vi "TestData_MySQL_OP-TEST.vi"(8 "error in (no error)":errorcluster, 10 "SQL File":path, 11 "Connection In":refnum<k7>) -> (0 "error out":errorcluster, 2 "ok?":bool, 3 "ADODB._Connection Out":refnum<k7>)   [LabVIEW 2012, in "Lib_UEL.ATE.lvlib" / "Lib_TestData.lvlib"]
uses:
  Lib_TestData.lvlib
  <vilib>/Utility/file.llb/Read From Spreadsheet File (string).vi
  <vilib>/Utility/file.llb/Write To Spreadsheet File (string).vi
panel:
  out "数组":i32[](array[numeric])
  out "Data":string[][](array[string])
  in  "Output Failed Record":bool
  out "Modified?":bool
  in  "Comment Signal":string
  out "Result":T1
  in  "TXT File In":path
  in  "ConnectionString":T2={"IP"="localhost", "Port"="3306", "DataBase"="uel_te", "User"="root", "Password"="alpha130723"}
  out "结果字符串":string
  # "功能描述:\n- 批量插入文本数据记录到数据库.\n- 插入成功的记录, 记录前以';'注释\n- 插入失败的记录, 不注释\n- 已注释的记录, 不会进行插入数据的操作.\n- Output Failed Record开关: 失败的记录是否导出到一个单独的文件, 打开后, 输出到文件名: 原文件名+FailInsert+Date."
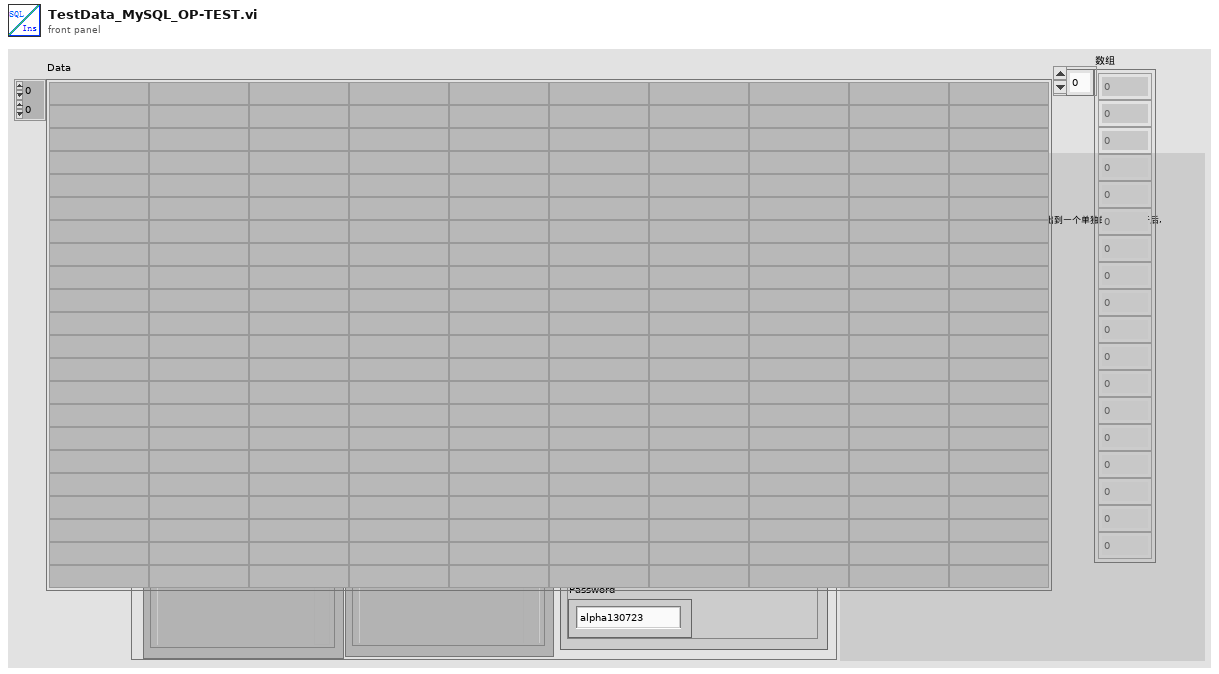
[diagram p1: front panel]
types:
  T1 = cluster{"Total":u32, "NG":u32, "OK":u32, "Ignore":u32}
  T2 = cluster{"IP":string, "Port":string, "DataBase":string, "User":string, "Password":string}
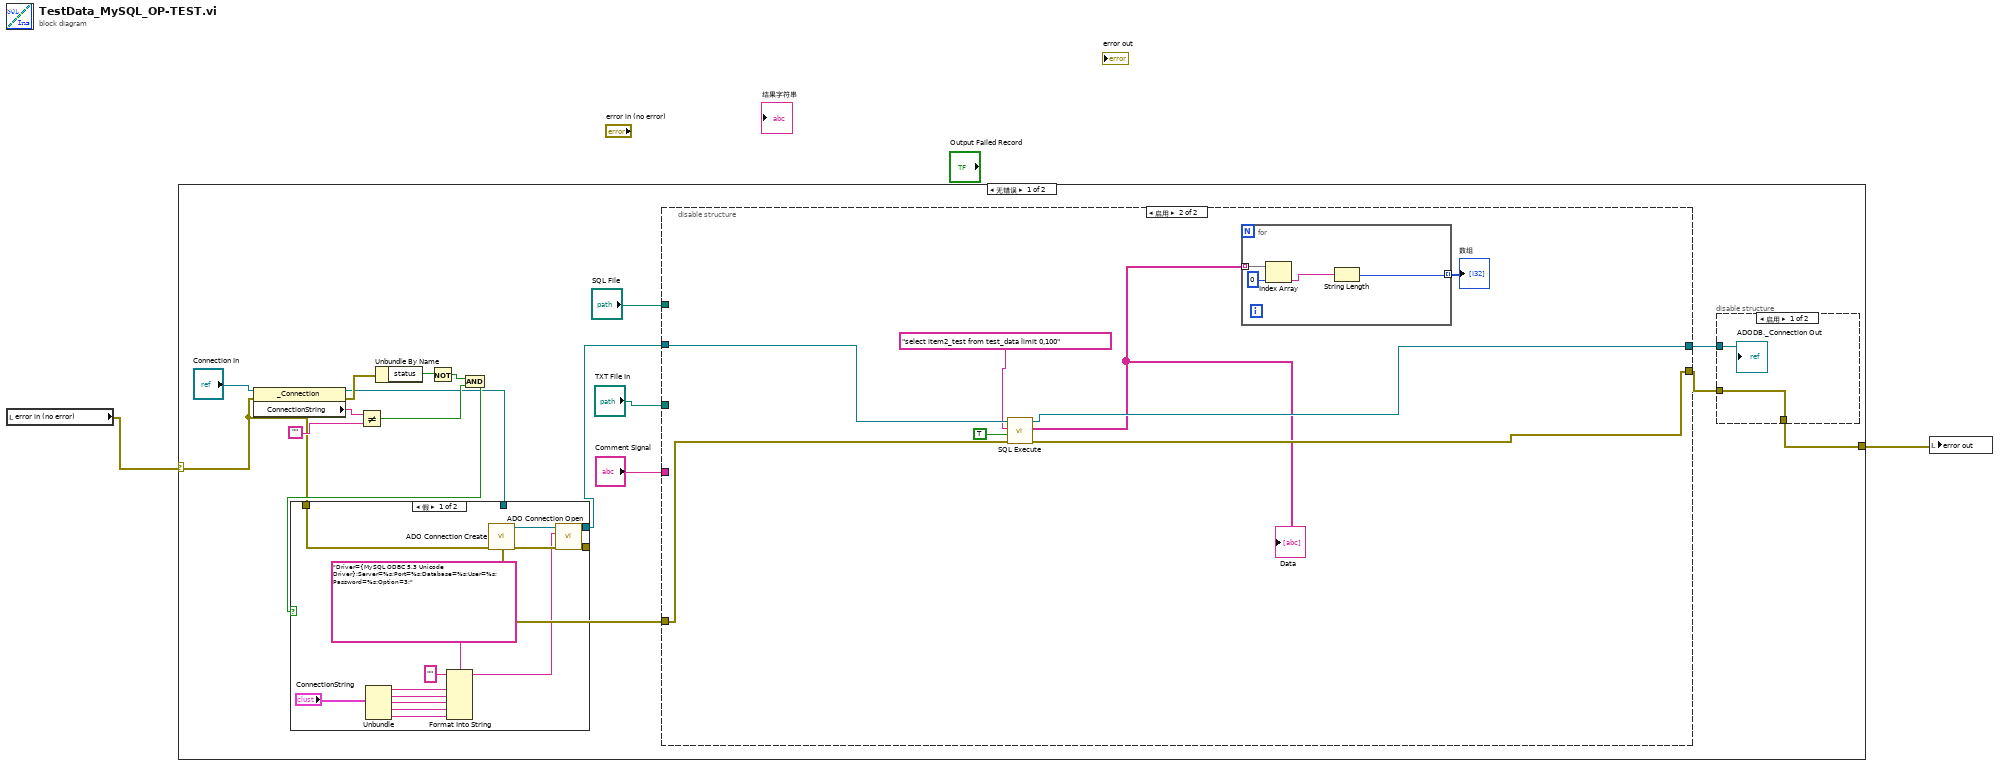
[diagram p0: block diagram]
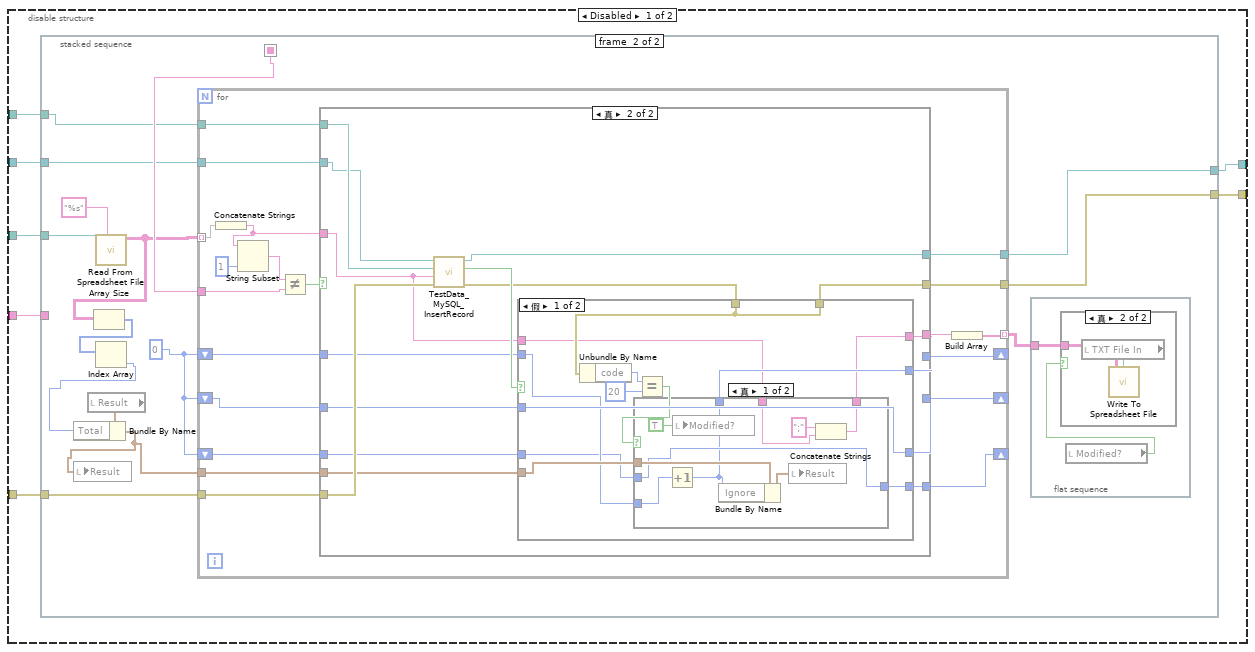
[diagram p2: hidden frame]
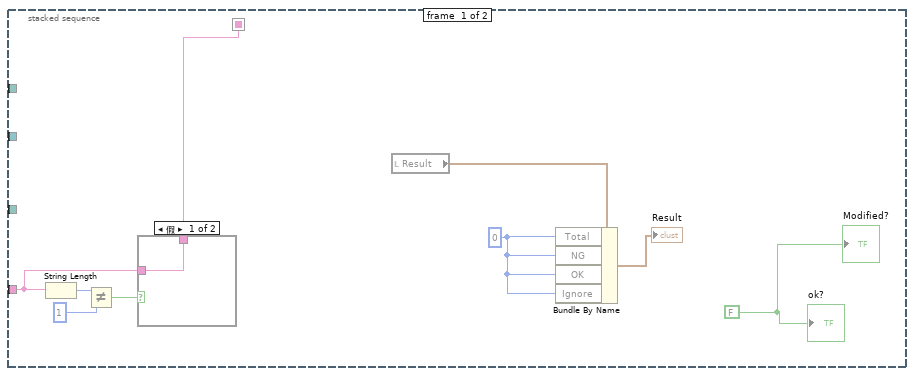
[diagram p3: hidden frame]
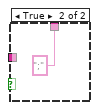
[diagram p4: hidden frame]
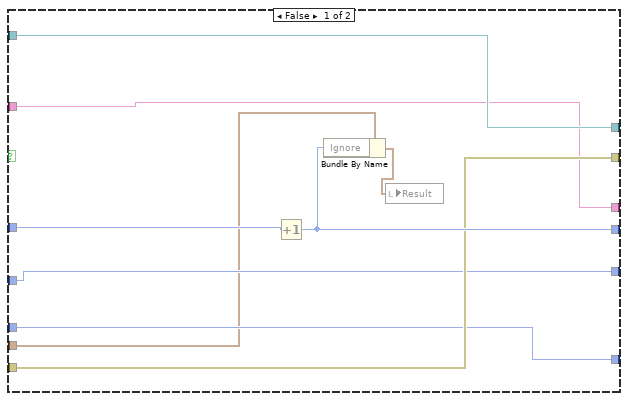
[diagram p6: hidden frame]
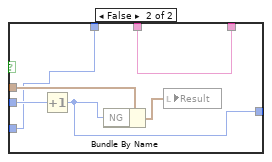
[diagram p7: hidden frame]
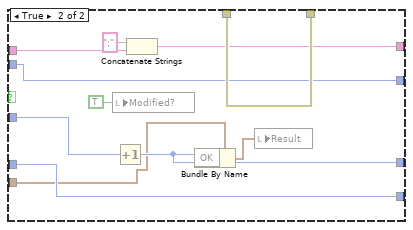
[diagram p8: hidden frame]
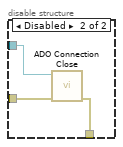
[diagram p10: hidden frame]
diagram:
  n1 = local read "error in (no error)"() -> (w1:errorcluster)
  n2 = case shown="无错误" w1 {
    selector: w1 -> [w3 w174]
    tunnel: [w4 w174] -> w2
    frame No Error {
      n3 = property class="_Connection"(reference="Connection In", error in=w3) -> (reference out=w6:refnum<k7>, error out=w11:errorcluster, "ConnectionString"=w13:string)
      n4 = Not Equal?(x=w13, y="") -> (x != y?=w8:bool)
      n5 = Unbundle By Name(w11) -> ("status"=w10:bool)
      n6 = Not(x=w10) -> (.not. x?=w9:bool)
      n7 = And(x=w9, y=w8) -> (x .and. y?=w7:bool)
      n8 = case shown="假" w7 {
        tunnel: [w166 w168] -> w15
        tunnel: w6 -> [_ w168]
        tunnel: w3 -> [w154 w167]
        tunnel: [w153 w167] -> w5
        frame False {
          n9 = Unbundle("ConnectionString") -> ("IP"=w158:string, "Port"=w159:string, "DataBase"=w160:string, "User"=w161:string, "Password"=w162:string)
          n10 = Format Into String(format string="Driver={MySQL ODBC 5.3 Unicode Driver};Server=%s;Port=%s;Database=%s;User=%s; Password=%s;Option=3;" ("格式字符串"), initial string="" ("初始字符串"), w158, w159, w160, w161, w162) -> (resulting string=w164:string)  [unwired: 1 in, 1 out]
          n11 = call <userlib>:"ADO Connection Create.vi"("error in (no error)"=w154) -> ("error out"=w163:errorcluster, "ADODB._Connection Out"=w165:refnum<k7>)  [unwired: 9 in]
          n12 = call <userlib>:"ADO Connection Open.vi"("error in (no error)"=w163, "ConnectionString"=w164, "ADODB._Connection In"=w165) -> ("error out"=w153:errorcluster, "ADODB._Connection Out"=w166:refnum<k7>)  [unwired: 7 in]
        }
        frame True {
        }
      }
      n13 = disable-structure shown="启用" {
        disable-tunnel: [w27 w145] -> w20
        disable-tunnel: "SQL File" -> [w26 _]
        disable-tunnel: "TXT File In" -> [w25 _]
        disable-tunnel: "Comment Signal" -> [w24 _]
        disable-tunnel: [w23 w144] -> w16
        disable-tunnel: w15 -> [w22 w147]
        disable-tunnel: w5 -> [w21 w146]
        frame Disabled {
          n14 = stacked-sequence {
            seq-local: [w33 _] -> [_ w51]
            tunnel: w21 -> [_ w47]
            tunnel: [_ w44] -> w27
            tunnel: [_ w45] -> w23
            tunnel: w26 -> [_ w46]
            tunnel: w25 -> [_ w53]
            tunnel: w24 -> [w32 _]
            tunnel: w22 -> [_ w43]
            frame #0 {
              w29 = u32 0 ("Total")
              w28 = FALSE ("ok?")
              n15 = String Length(string=w32) -> (length=w36:i32)
              n16 = Not Equal?(x=w36, y=1) -> (x != y?=w34:bool)
              n17 = case shown="假" w34 {
                tunnel: [w37 ";"] -> w33
                tunnel: w32 -> [w37 _]
                frame False {
                }
                frame True {
                }
              }
              n18 = local read "Result"() -> (w31:T1)
              n19 = Bundle By Name(cluster=w31, "Total"=w29, "NG"=w29, "OK"=w29, "Ignore"=w29) -> (→"Result":T1)
              "ok?" <- w28
              "Modified?" <- w28
            }
            frame #1 {
              w48 = 0
              n20 = local read "Result"() -> (w42:T1)
              n21 = call-poly <vilib>:"Read From Spreadsheet File.vi"("format (%s)"="%s", "file path (dialog if empty)"=w53) -> ("all rows"=w50:string[][])  [unwired: 5 in, 4 out]
              n22 = Array Size(array=w50) -> (size(s)=w49:i32[])
              n23 = Index Array(array=w49) -> (element=w41:i32)  [unwired: 1 in]
              n24 = Bundle By Name(cluster=w42, "Total"=w41) -> (w40:T1)
              n25 = local write "Result"(w40) -> ()
              n26 = for {
                tunnel: w50 -> [w77] mode=indexing
                tunnel: w51 -> [w74]
                shift-right: [w71] -> _
                shift-left: w48 -> [w72]
                shift-right: [w63] -> _
                shift-left: w48 -> [w64]
                shift-right: [w62] -> _
                shift-left: w48 -> [w61]
                tunnel: w47 -> [w70]
                tunnel: w46 -> [w68]
                tunnel: [w67] -> w45
                tunnel: [w66] -> w44
                tunnel: w43 -> [w65]
                tunnel: w40 -> [w60]
                tunnel: [w58] -> w39 mode=indexing
                n27 = Concatenate Strings(w77) -> (w69:string)
                n28 = String Subset(string=w69, length (rest)=1 ("长度（剩余）")) -> (substring=w75:string)  [unwired: 1 in]
                n29 = Not Equal?(x=w75, y=w74) -> (x != y?=w73:bool)
                n30 = case shown="真" w73 {
                  tunnel: w72 -> [w86 w90]
                  tunnel: [w85 w89] -> w71
                  tunnel: w70 -> [w83 w102]
                  tunnel: w69 -> [w78 w88]
                  tunnel: w68 -> [_ w101]
                  tunnel: [w83 w92] -> w67
                  tunnel: [w82 w100] -> w66
                  tunnel: w65 -> [w82 w99]
                  tunnel: w64 -> [w81 w97]
                  tunnel: [w81 w96] -> w63
                  tunnel: [w80 w95] -> w62
                  tunnel: w61 -> [w80 w94]
                  tunnel: w60 -> [w79 w93]
                  tunnel: [w78 w87] -> w59
                  frame False {
                    n31 = Increment(x=w86) -> (x+1=w85:i32)
                    n32 = Bundle By Name(cluster=w79, "Ignore"=w85) -> (w84:T1)
                    n33 = local write "Result"(w84) -> ()
                  }
                  frame True {
                    n34 = call "TestData_MySQL_InsertRecord.vi"("error in (no error)"=w102, "data_input"=w88, "SQL File"=w101, "Connection In"=w99) -> ("error out"=w91:errorcluster, "ok?"=w98:bool, "ADODB._Connection Out"=w100:refnum<k7>)  [unwired: 5 in]
                    n35 = case shown="假" w98 {
                      tunnel: w97 -> [w114 w139]
                      tunnel: [w114 w138] -> w96
                      tunnel: [w113 w137] -> w95
                      tunnel: w94 -> [w106 w137]
                      tunnel: w93 -> [w112 w136]
                      tunnel: [w111 w135] -> w92
                      tunnel: w91 -> [w111 w135]
                      tunnel: w90 -> [w107 w134]
                      tunnel: [w105 w134] -> w89
                      tunnel: w88 -> [w104 w133]
                      tunnel: [w103 w131] -> w87
                      frame False {
                        n36 = Unbundle By Name(w111) -> ("code"=w110:i32)
                        n37 = Equal?(x=w110, y=20) -> (x = y?=w108:bool)
                        n38 = case shown="真" w108 {
                          tunnel: w106 -> [w120 w128]
                          tunnel: [w120 w127] -> w113
                          tunnel: w112 -> [w122 w126]
                          tunnel: w107 -> [w121 w125]
                          tunnel: [w119 w125] -> w105
                          tunnel: w104 -> [w117 w124]
                          tunnel: [w116 w124] -> w103
                          frame True {
                            n39 = Increment(x=w121) -> (x+1=w119:i32)
                            n40 = local write "Modified?"(TRUE ("Modified?")) -> ()
                            n41 = Bundle By Name(cluster=w122, "Ignore"=w119) -> (w123:T1)
                            n42 = local write "Result"(w123) -> ()
                            n43 = Concatenate Strings(";" ("字符串"), w117) -> (w116:string)
                          }
                          frame False {
                            n44 = Increment(x=w128) -> (x+1=w127:i32)
                            n45 = Bundle By Name(cluster=w126, "NG"=w127) -> (w129:T1)
                            n46 = local write "Result"(w129) -> ()
                          }
                        }
                      }
                      frame True {
                        n47 = local write "Modified?"(TRUE ("Modified?")) -> ()
                        n48 = Increment(x=w139) -> (x+1=w138:i32)
                        n49 = Concatenate Strings(";" ("字符串"), w133) -> (w131:string)
                        n50 = Bundle By Name(cluster=w136, "OK"=w138) -> (w140:T1)
                        n51 = local write "Result"(w140) -> ()
                      }
                    }
                  }
                }
                n52 = Build Array(w59) -> (w58:string[])
              }
              n53 = flat-sequence {
                tunnel: w39 -> [w55]
                frame #0 {
                  n54 = local read "Modified?"() -> (w54:bool)
                  n55 = case shown="真" w54 {
                    tunnel: w55 -> [_ w56]
                    frame False {
                    }
                    frame True {
                      n56 = local read "TXT File In"() -> (w57:path)
                      n57 = call-poly <vilib>:"Write To Spreadsheet File.vi"("2D data"=w56, "file path (dialog if empty)"=w57) -> ()  [unwired: 6 in, 1 out]
                    }
                  }
                }
              }
            }
          }
        }
        frame Enabled {
          n58 = call <userlib>:"SQL Execute.vi"("error in (no error)"=w146, "Return Data (T)"=TRUE, "Command Text"="select item2_test from test_data limit 0,100" ("格式字符串"), "ADODB._Connection In"=w147) -> ("error out"=w144:errorcluster, "Data"=w142:string[][], "ADODB._Connection Out"=w145:refnum<k7>)  [unwired: 4 in, 1 out]
          "Data" <- w142
          n59 = for {
            tunnel: w142 -> [w152] mode=indexing
            tunnel: [w149] -> w141 mode=indexing
            n60 = Index Array(array=w152, index=0 ("索引")) -> (element=w150:string)
            n61 = String Length(string=w150) -> (length=w149:i32)
          }
          "数组" <- w141
        }
      }
      n62 = disable-structure shown="启用" {
        disable-tunnel: w20 -> [w170 w173]
        disable-tunnel: w16 -> [w169 w172]
        disable-tunnel: [w169 w171] -> w4
        frame Enabled {
          "ADODB._Connection Out" <- w170
        }
        frame Disabled {
          n63 = call <userlib>:"ADO Connection Close.vi"("error in (no error)"=w172, "ADODB._Connection In"=w173) -> ("error out"=w171:errorcluster)  [unwired: 8 in, 1 out]
        }
      }
    }
    frame Error {
    }
  }
  n64 = local write "error out"(w2) -> ()
